vi "Get IPs.vi"(8 "error in":errorcluster, 10 "File Name":string="InstrumentsConfig.ini", 11 "path":path=path "C:/TDS/t230054-rf-mezz-fct-main/Configuration") -> (0 "error out":errorcluster, 2 "VISA Cluster":T1={"[PS1]"="PS_Rigol_1", "[PS2]"="PS_Rigol_2", "[PS3]"="PS_Rigol_3", "[PS4]"="PS_Rigol_4", "[PowerMeter]"="PowerMeter", "[SigGen]"="TCPIP0::192.168.10.31::INSTR", "[RF_Switch]"="TCPIP0::192.168.10.32::INSTR"}, 3 "IP Cluster":T2={"[TrenNet1]"="192.168.10.11", "[TrenNet2]"="192.168.10.12", "[TrenNet3]"="192.168.10.13", "[TrenNet4]"="192.168.10.14", "[PS1]"="192.168.10.21", "[PS2]"="192.168.10.22", "[PS3]"="192.168.10.23", "[PS4]"="192.168.10.24", "[PowerMeter]"="192.168.10.30", "[SigGen]"="192.168.10.31", "[RF_Switch]"="192.168.10.32", "[Numato]"="COM3", "[UUT1]"="192.168.10.41", "[UUT2]"="192.168.10.42", "[UUT3]"="192.168.10.43", "[UUT4]"="192.168.10.44"})   [LabVIEW 2023]
uses:
  <vilib>/Utility/config.llb/Read Key (String).vi
  <vilib>/Utility/config.llb/NI_LVConfig.lvlib
panel:
  in  "Instruments VISA Array":string[](array[string])=["PS1", "PS2", "PS3", "PS4", "PowerMeter", "SigGen", "RF Switch"]
  in  "Instruments IP Array":string[](array[string])=["TrenNet1", "TrenNet2", "TrenNet3", "TrenNet4", "PS1", "PS2", "PS3", "PS4", "PowerMeter", "SigGen", "RF Switch", "Numato", "UUT1", "UUT2", "UUT3", "UUT4"]
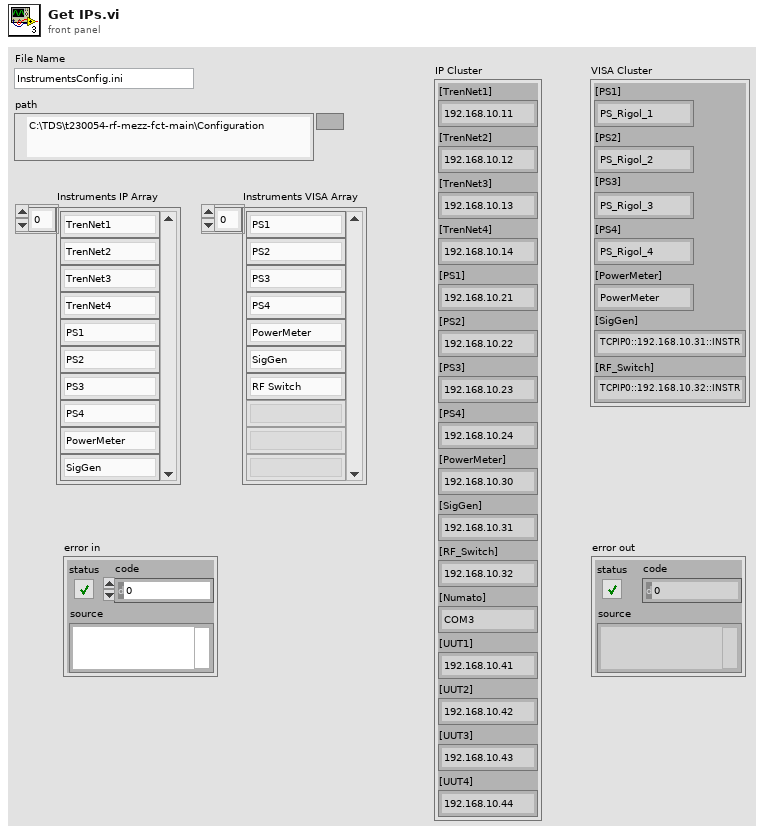
[diagram p1: front panel]
types:
  T1 = cluster{"[PS1]":string, "[PS2]":string, "[PS3]":string, "[PS4]":string, "[PowerMeter]":string, "[SigGen]":string, "[RF_Switch]":string}
  T2 = cluster{"[TrenNet1]":string, "[TrenNet2]":string, "[TrenNet3]":string, "[TrenNet4]":string, "[PS1]":string, "[PS2]":string, "[PS3]":string, "[PS4]":string, "[PowerMeter]":string, "[SigGen]":string, "[RF_Switch]":string, "[Numato]":string, "[UUT1]":string, "[UUT2]":string, "[UUT3]":string, "[UUT4]":string}
  T3 = cluster{"[0]":string, "[1]":string, "[2]":string, "[3]":string, "[4]":string, "[5]":string, "[6]":string}
  T4 = cluster{"[0]":string, "[1]":string, "[2]":string, "[3]":string, "[4]":string, "[5]":string, "[6]":string, "[7]":string, "[8]":string, "[9]":string, "[10]":string, "[11]":string, "[12]":string, "[13]":string, "[14]":string, "[15]":string}
  T5 = typedef "NI_LVConfig.lvlib/Config Data RefNum.ctl" = refnum<k1>
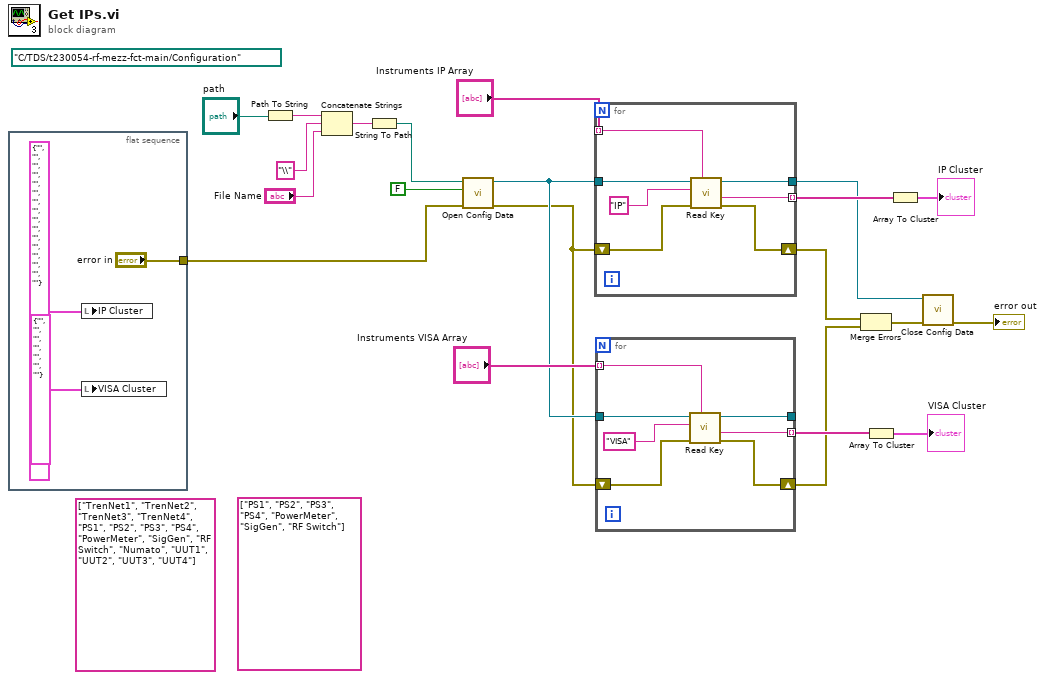
[diagram p0: block diagram]
diagram:
  (unwired) string[] ["PS1", "PS2", "PS3", "PS4", "PowerMeter", "SigGen", "RF Switch"] ("Instruments VISA Array")
  (unwired) string[] ["TrenNet1", "TrenNet2", "TrenNet3", "TrenNet4", "PS1", "PS2", "PS3", "PS4", "PowerMeter", "SigGen", "RF Switch", "Numato", "UUT1", "UUT2", "UUT3", "UUT4"] ("Instruments IP Array")
  (unwired) path "C:/TDS/t230054-rf-mezz-fct-main/Configuration"
  n1 = flat-sequence {
    tunnel: ["error in"] -> w3
    frame #0 {
      n2 = local write "IP Cluster"(T4 {"[0]"="", "[1]"="", "[2]"="", "[3]"="", "[4]"="", "[5]"="", "[6]"="", "[7]"="", "[8]"="", "[9]"="", "[10]"="", "[11]"="", "[12]"="", "[13]"="", "[14]"="", "[15]"=""} ("IP Cluster")) -> ()
      n3 = local write "VISA Cluster"(T3 {"[0]"="", "[1]"="", "[2]"="", "[3]"="", "[4]"="", "[5]"="", "[6]"=""} ("VISA Cluster")) -> ()
    }
  }
  n4 = Path To String(path="path") -> (string=w18:string)
  n5 = Concatenate Strings(w18, "\\" ("string"), "File Name") -> (w21:string)
  n6 = String To Path(string=w21) -> (path=w1:path)
  n7 = call <vilib>:"Open Config Data.vi"("error in (no error)"=w3, "create file if necessary (T)"=FALSE, "configuration file path"=w1) -> ("error out"=w11:errorcluster, "refnum"=w12:T5)  [unwired: 6 in, 1 out]
  n8 = for {
    tunnel: "Instruments IP Array" -> [w31] mode=indexing
    tunnel: w12 -> [w30]
    tunnel: [w28] -> w5
    shift-right: [w26] -> w8
    shift-left: w11 -> [w27]
    tunnel: [w25] -> w15 mode=indexing
    n9 = call-poly <vilib>:"Read Key.vi"("section"=w31, "error in (no error)"=w27, "key"="IP", "refnum"=w30) -> ("error out"=w26:errorcluster, "value"=w25:string, "refnum out"=w28:T5)  [unwired: 4 in, 1 out]
  }
  n10 = for {
    tunnel: "Instruments VISA Array" -> [w38] mode=indexing
    tunnel: w12 -> [w37]
    tunnel: [w35] -> _
    shift-right: [w33] -> w7
    shift-left: w11 -> [w34]
    tunnel: [w32] -> w10 mode=indexing
    n11 = call-poly <vilib>:"Read Key.vi"("section"=w38, "error in (no error)"=w34, "key"="VISA", "refnum"=w37) -> ("error out"=w33:errorcluster, "value"=w32:string, "refnum out"=w35:T5)  [unwired: 4 in, 1 out]
  }
  n12 = Merge Errors(w8, w7) -> (w6:errorcluster)
  n13 = Array To Cluster(array=w10) -> (cluster=→"VISA Cluster":T3)
  n14 = Array To Cluster(array=w15) -> (cluster=→"IP Cluster":T4)
  n15 = call <vilib>:"Close Config Data.vi"("error in (no error)"=w6, "refnum"=w5) -> ("error out"=→"error out":errorcluster)  [unwired: 8 in, 1 out]
